vi "dbase string to variant.vi"(8 "error in (no error)":errorcluster, 11 "String":string) -> (0 "error out":errorcluster, 3 "Variant":variant)   [LabVIEW 2017]
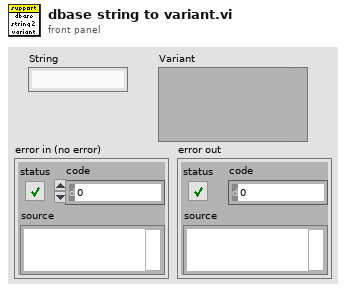
[diagram p1: front panel]
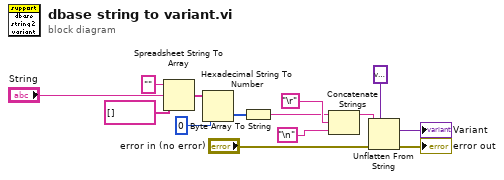
[diagram p0: block diagram]
diagram:
  n1 = Spreadsheet String To Array(format string="", spreadsheet string="String", array type (2D Dbl)=string[] [] ("hex integer string")) -> (array=w8:string[])  [unwired: 1 in]
  n2 = Hexadecimal String To Number(string=w8, default (0uL)=u8 0) -> (number=w6:u8[])  [unwired: 1 in, 1 out]
  n3 = Byte Array To String(unsigned byte array=w6) -> (string=w1:string)
  n4 = Concatenate Strings(w1, "\r", "\n") -> ()  [unwired: 1 out]
  n5 = Unflatten From String(type=variant ("Variant"), binary string=w1, error in (no error)="error in (no error)") -> (value=→"Variant":variant, error out=→"error out":errorcluster)  [unwired: 2 in, 1 out]
